vi "Stop Core.vi"(10 "final error code":i32, 11 "BNT_XtGraph in":refnum<class "BNT_XtGraph.lvclass">) -> (3 "BNT_XtGraph out":refnum<class "BNT_XtGraph.lvclass">)   [LabVIEW 2018, in "BNT_XtGraph.lvlib" / "BNT_XtGraph.lvclass"]
doc: "(<B>Filename</B>: Actor Framework.lvlib:Actor.lvclass:Stop Core.vi)\n\nDefines what the actor does before it stops. Use the <B>final error code</B> input to determine whether the actor shut down in response to an error.\n\nBy default, this method does nothing. A descendant class may override it to define behavior, such as shutting down any processes the actor initiated in its override of the Actor Core method."
uses:
  BNT_XtGraph.lvclass
  BNT_XtGraph.lvclass/BNT_XtGraph.ctl
  CSPP_Core/Actors/CSPP_BaseActor/CSPP_BaseActor.lvclass
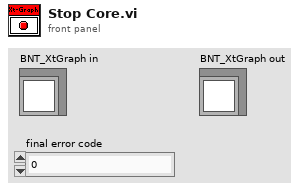
[diagram p1: front panel]
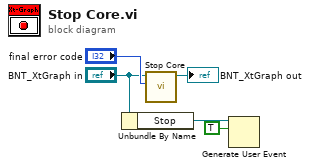
[diagram p0: block diagram]
diagram:
  n1 = Unbundle By Name("BNT_XtGraph in") -> ("Stop"=w2:refnum<user-event>)
  n2 = call-parent "Stop Core.vi"("final error code"="final error code", "CSPP_BaseActor in"="BNT_XtGraph in") -> ("CSPP_BaseActor out"=→"BNT_XtGraph out":refnum<class "BNT_XtGraph.lvclass">)  [unwired: 9 in]
  n3 = Generate User Event(user event=w2, event data cluster=TRUE ("event data")) -> ()  [unwired: 2 in, 2 out]
